vi "event_structure.vi"() -> ()   [LabVIEW 2019]
panel:
  out "element":i32
  in  "stop":bool
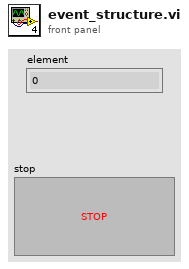
[diagram p1: front panel]
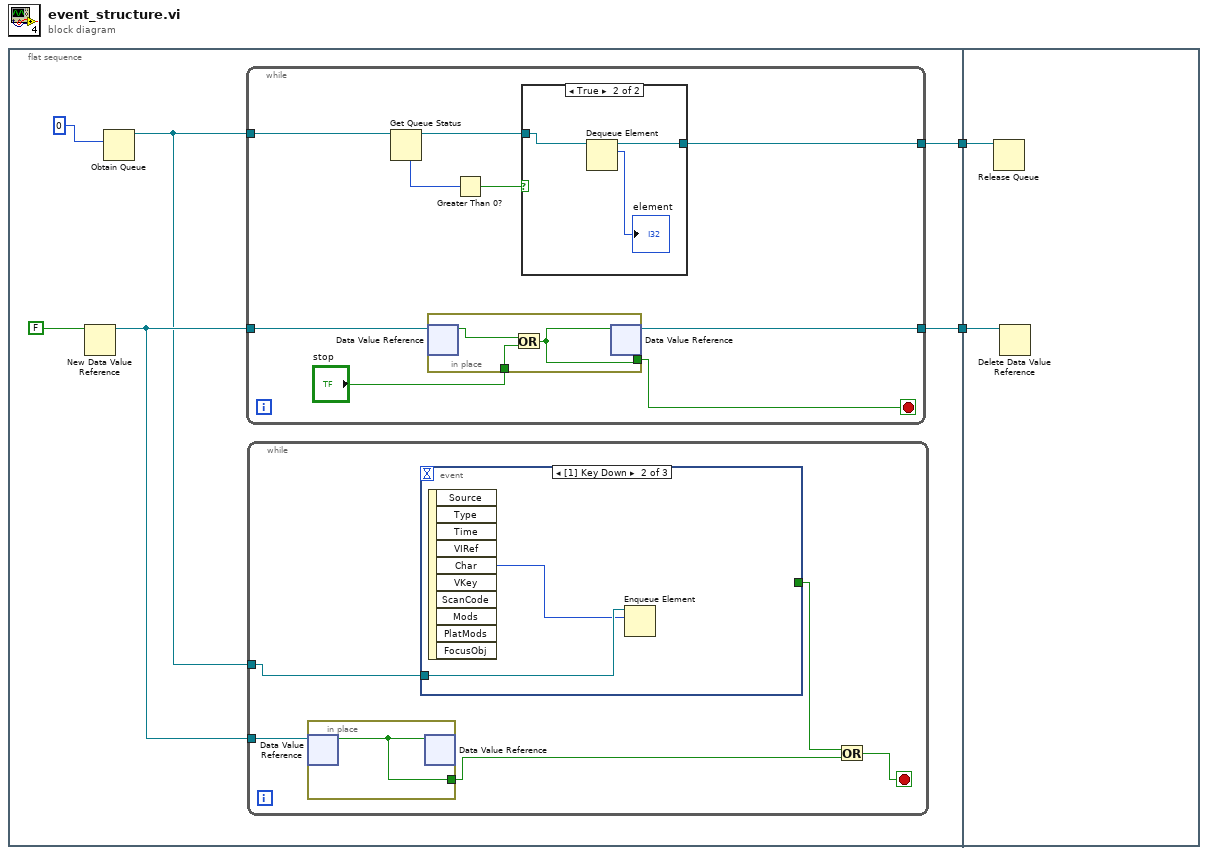
[diagram p0: block diagram]
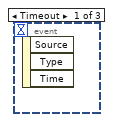
[diagram p3: hidden frame]
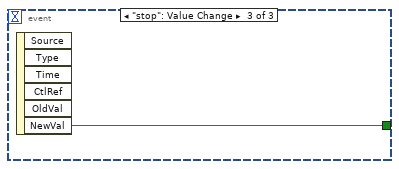
[diagram p4: hidden frame]
diagram:
  n1 = flat-sequence {
    tunnel: [w6] -> w2
    tunnel: [w3] -> w1
    tunnel: w2 -> [w34]
    tunnel: w1 -> [w35]
    frame #0 {
      n2 = New Data Value Reference(data value=FALSE) -> (data value reference=w7:refnum<data-value>)  [unwired: 1 in, 1 out]
      n3 = Obtain Queue(element data type=0) -> (queue out=w4:refnum<queue>)  [unwired: 4 in, 2 out]
      n4 = while {
        tunnel: w7 -> [w17]
        tunnel: [w15] -> w6
        tunnel: w4 -> [w13]
        tunnel: [w9] -> w3
        stop <- w14 stop-if-true
        n5 = Get Queue Status(queue=w13) -> (queue out=w10:refnum<queue>, # elements in queue=w12:i32)  [unwired: 2 in, 6 out]
        n6 = in-place {
          in-place-border: "stop" -> [w23]
          in-place-border: [w22] -> w14
          n7 = in-place-dvr #1(w17) -> (w24:bool)  [unwired: 1 out]
          n8 = Or(x=w24, y=w23) -> (x .or. y?=w22:bool)
          n9 = in-place-dvr #1(w22) -> (w15:refnum<data-value>)  [unwired: 1 out]
        }
        n10 = Greater Than 0?(x=w12) -> (x > 0?=w11:bool)
        n11 = case shown="True" w11 {
          tunnel: w10 -> [w18 w21]
          tunnel: [w18 w19] -> w9
          frame False {
          }
          frame True {
            n12 = Dequeue Element(queue=w21) -> (queue out=w19:refnum<queue>, element=→"element":i32)  [unwired: 2 in, 2 out]
          }
        }
      }
      n13 = while {
        tunnel: w7 -> [w29]
        tunnel: w4 -> [w28]
        stop <- w25 stop-if-true
        n14 = in-place {
          in-place-border: [w30] -> w26
          n15 = in-place-dvr #2(w29) -> (w30:bool)  [unwired: 1 out]
          n16 = in-place-dvr #2(w30) -> ()  [unwired: 2 out]
        }
        n17 = event shown="[1] Key Down" {
          selector: _ -> [_ _ _]
          dyn-events: _ -> [_ _ _]
          timeout: _ -> [_ _ _]
          tunnel: w28 -> [_ w32 _]
          tunnel: [_ _ w33] -> w27
          event Timeout {
            n18 = event-data() -> ()  [unwired: 1 in, 3 out]
          }
          event Key Down {
            n19 = event-data() -> ("Char"=w31:i16)  [unwired: 1 in, 9 out]
            n20 = Enqueue Element(queue=w32, element=w31) -> ()  [unwired: 2 in, 3 out]
          }
          event "stop": Value Change {
            n21 = event-data() -> ("NewVal"=w33:bool)  [unwired: 1 in, 5 out]
          }
        }
        n22 = Or(x=w27, y=w26) -> (x .or. y?=w25:bool)
      }
    }
    frame #1 {
      n23 = Release Queue(queue=w35) -> ()  [unwired: 2 in, 3 out]
      n24 = Delete Data Value Reference(data value reference=w34) -> ()  [unwired: 1 in, 2 out]
    }
  }
